vi "DrawGcylinders.vi"(1 "Object in":refnum<vi>, 3 "Color":T1={"Red"=1.0, "Green"=0.0, "Blue"=0.0, "Alpha"=1.0}, 4 "contents":string) -> (0 "Object out":refnum<vi>, 2 "remaining":string)   [LabVIEW 2010]
uses:
  <vilib>/picture/3D Picture Control/NI_3D Picture Control.lvlib
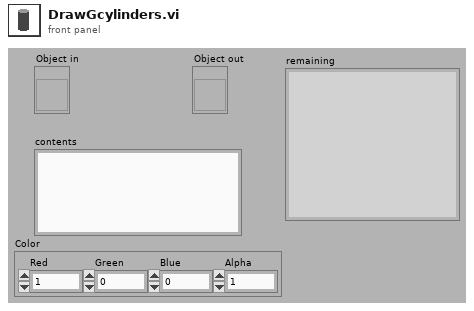
[diagram p1: front panel]
types:
  T1 = cluster{"Red":sgl, "Green":sgl, "Blue":sgl, "Alpha":sgl}
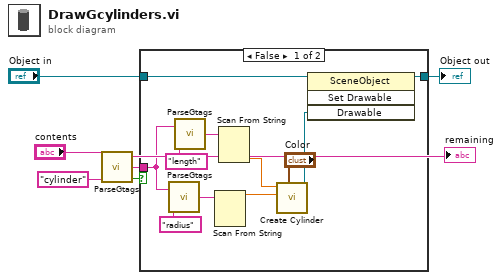
[diagram p0: block diagram]
diagram:
  n1 = call "ParseGtags.vi"("tag"="cylinder", "urdf in"="contents") -> ("not found"=w4:bool, "contents"=w5:string, "urdf out"=→"remaining":string)  [unwired: 1 out]
  n2 = case shown="False" w4 {
    tunnel: w5 -> [w16 _]
    tunnel: "Object in" -> [w12 w19]
    tunnel: [w11 w19] -> w7
    frame False {
      n3 = call "ParseGtags.vi"("tag"="radius", "urdf in"=w16) -> ("contents"=w14:string)  [unwired: 3 out]
      n4 = call "ParseGtags.vi"("tag"="length", "urdf in"=w16) -> ("contents"=w15:string)  [unwired: 3 out]
      n5 = Scan From String(input string=w14) -> (output 1=w13:dbl)  [unwired: 4 in, 3 out]
      n6 = Scan From String(input string=w15) -> (output 1=w8:dbl)  [unwired: 4 in, 3 out]
      n7 = call <vilib>:"Create Cylinder.vi"("Color"="Color", "Radius"=w13, "Height"=w8) -> ("New Cylinder Refnum"=w10:refnum<vi>)  [unwired: 7 in, 1 out]
      n8 = invoke class="SceneObject" method="Set Drawable"(reference=w12, "Drawable"=w10) -> (reference out=w11:refnum<vi>)  [unwired: 2 in, 3 out]
    }
    frame True {
    }
  }
  "Object out" <- w7
